vi "Read TCPClient.vi"(8 "error in (no error)":errorcluster, 11 "MonoClient in":refnum<class "MonoClientCommunicator.lvclass">) -> (0 "error out":errorcluster, 2 "TCPClient.lvclass":refnum<class "TCPClient.lvclass">, 3 "MonoClient out":refnum<class "MonoClientCommunicator.lvclass">)   [LabVIEW 2016, in "MonoClientCommunicator.lvclass"]
uses:
  MonoClientCommunicator.lvclass
  ts_labview_tcp/TCPClient/TCPClient.lvclass
  MonoClientCommunicator.lvclass/MonoClientCommunicator.ctl
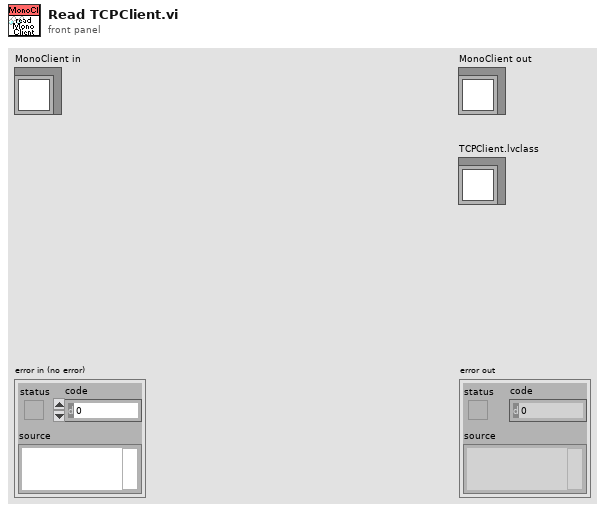
[diagram p1: front panel]
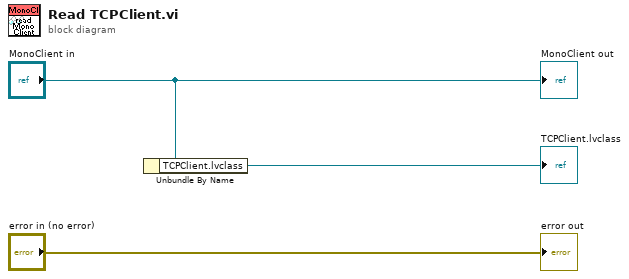
[diagram p0: block diagram]
diagram:
  n1 = Unbundle By Name("MonoClient in") -> ("TCPClient.lvclass"=→"TCPClient.lvclass":refnum<class "TCPClient.lvclass">)
  "error out" <- "error in (no error)"
  "MonoClient out" <- "MonoClient in"
